vi "RS 232 read_write.vi"() -> ()   [LabVIEW 2013]
panel:
  out "concatenated string":string
  in  "Data Field":string="*IDN?"
  out "read string":string
  in  "bytes to read":u32=5
  in  "read":bool=TRUE
  in  "flow control":u16(ring) items=["None"=0, "XON/XOFF"=1, "RTS/CTS"=2, "DTR/DSR"=4]
  in  "write":bool=TRUE
  in  "stop bits":u16(ring)=10 items=["1.0"=10, "1.5"=15, "2.0"=20]
  in  "parity":u16(ring) items=["None", "Odd", "Even", "Mark", "Space"]
  in  "data bits":u16=8 min=5 max=8 step=1
  in  "baud rate":u32=9600
  in  "VISA resource name":refnum<visa-resource-name>="COM1"
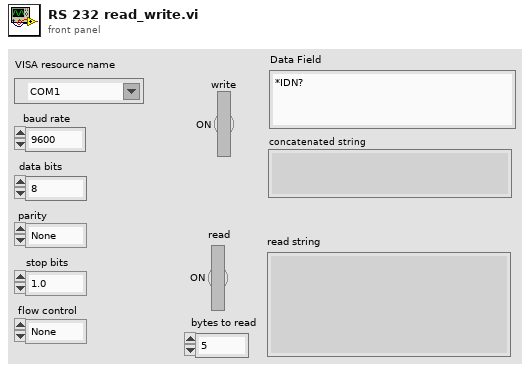
[diagram p1: front panel]
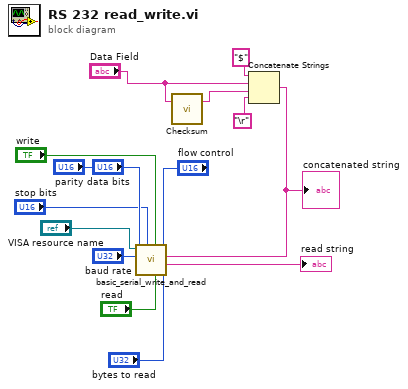
[diagram p0: block diagram]
diagram:
  n1 = call "Checksum.vi"("string to write"="Data Field") -> ("ASCII Output"=w10:string)  [unwired: 2 in]
  n2 = Concatenate Strings("$" ("string"), "Data Field", w10, "\r") -> (w12:string)
  "concatenated string" <- w12
  n3 = call "basic_serial_write_and_read.vi"("VISA resource name"="VISA resource name", "baud rate"="baud rate", "data bits"="data bits", "parity"="parity", "stop bits"="stop bits", "write"="write", "read"="read", "flow control"="flow control", "string to write"=w12, "bytes to read"="bytes to read") -> ("read string"=→"read string":string)
